vi "GE 5565PIORC.Close.vi"(8 "error in (no error)":errorcluster, 11 "GE 5565PIORC":refnum<class "GE 5565PIORC.lvclass">) -> (0 "error out":errorcluster)   [LabVIEW 2017]
uses:
  Source/GE 5565PIORC.lvclass
  Source/GE 5565PIORC.lvclass/GE 5565PIORC.ctl
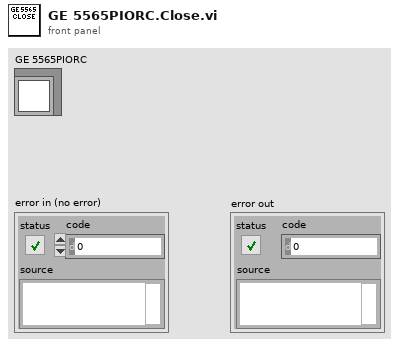
[diagram p1: front panel]
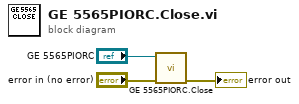
[diagram p0: block diagram]
diagram:
  n1 = call "GE 5565PIORC.Close.vi"("error in (no error)"="error in (no error)", "GE 5565PIORC in"="GE 5565PIORC") -> ("error out"=→"error out":errorcluster)  [unwired: 8 in, 1 out]
